vi "Get Projectile Atributes from ThreatGroupDetail.vi"(3 "error IN":errorcluster, 4 "ThreatDetail":refnum<vi>, 5 "ThreatGroup":refnum<vi>) -> (0 "error out":errorcluster, 2 "projectileAttribs":T1)   [LabVIEW 2015]
panel:
  out "queryStr":string
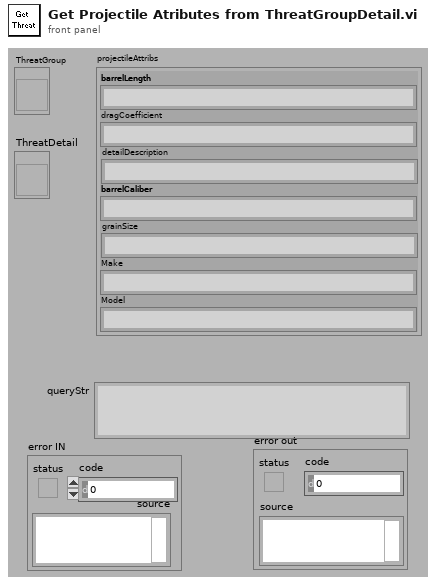
[diagram p1: front panel]
types:
  T1 = cluster{"barrelLength":string, "dragCoefficient":string, "detailDescription":string, "barrelCaliber":string, "grainSize":string, "Make":string, "Model":string}
  T2 = cluster{"[0]":string, "[1]":string, "[2]":string, "[3]":string, "[4]":string, "[5]":string, "[6]":string}
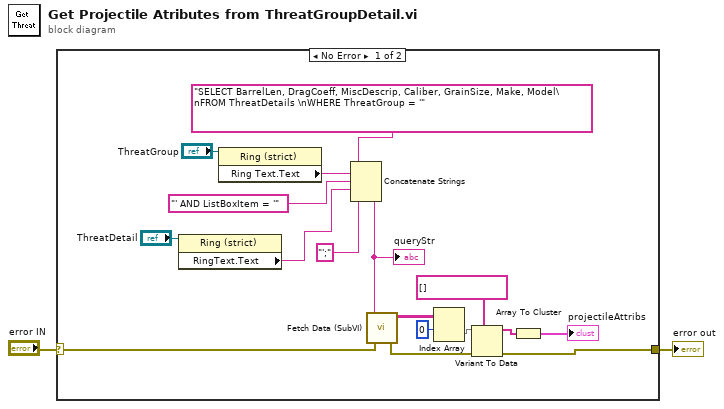
[diagram p0: block diagram]
diagram:
  n1 = case shown="No Error" "error IN" {
    selector: "error IN" -> [w8 w20]
    tunnel: [w6 w20] -> w1
    frame No Error {
      n2 = property on="Property Node" class="Ring (strict)"(reference="ThreatDetail") -> ("RingText.Text"=w3:string)  [unwired: 1 in, 2 out]
      n3 = property on="Property Node" class="Ring (strict)"(reference="ThreatGroup") -> ("Ring Text.Text"=w17:string)  [unwired: 1 in, 2 out]
      n4 = Concatenate Strings("SELECT BarrelLen, DragCoeff, MiscDescrip, Caliber, GrainSize, Make, Model\nFROM ThreatDetails \nWHERE ThreatGroup = '", w17, "' AND ListBoxItem = '" ("string"), w3, "';" ("string")) -> (w9:string)
      "queryStr" <- w9
      n5 = call "Fetch Data (SubVI).vi"("error IN"=w8, "query string"=w9) -> ("error OUT"=w7:errorcluster, "recordset data"=w19:string[][])  [unwired: 4 out]
      n6 = Index Array(array=w19, index (row)=0 ("disabled index (col)")) -> (element=w13:string[])  [unwired: 1 in]
      n7 = Variant To Data(error in=w7, type=string[] [], Variant=w13) -> (data=w11:string[], error out=w6:errorcluster)
      n8 = Array To Cluster(array=w11) -> (cluster=→"projectileAttribs":T2)
    }
    frame Error {
    }
  }
  "error out" <- w1
